vi "Configure Measurement.vi"(0 "Supply Handle in":refnum<k15>, 1 "Active Channel":string, 5 "Supply Measurement Settings":T1={"Measure When Mode"=enum."On Measure Trigger", "Sense Mode"=enum."Local", "Measurement Trigger Terminal"="PXI_Trig0", "Measurement Mode"=enum."Single Point", "Measurement Time (s)"=0.001} {"Measurement Time (s)" format="%#_13p"}, 11 "error in (no error)":errorcluster) -> (4 "Supply Handle out":refnum<k15>, 15 "error out":errorcluster)   [LabVIEW 2018, in "Supply.lvlib"]
uses:
  Supply.lvlib
  Typedefs/Measurement Configuration.ctl
  <instrlib>/niDCPower/nidcpower.llb/niDCPower Configure Digital Edge Measure Trigger.vi
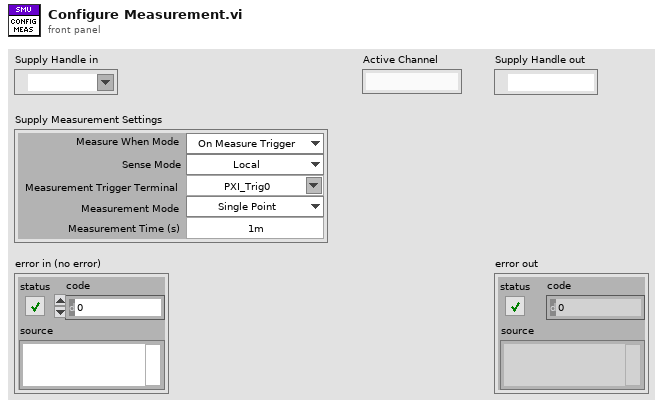
[diagram p1: front panel]
types:
  T1 = typedef "Supply.lvlib/Measurement Configuration.ctl" = cluster{"Measure When Mode":enum16{"Automatically after Source Complete", "On Demand", "On Measure Trigger"}, "Sense Mode":enum16{"Local", "Remote"}, "Measurement Trigger Terminal":string, "Measurement Mode":enum16{"Single Point", "Record"}, "Measurement Time (s)":dbl}
  T2 = enum16{"Automatically after Source Complete", "On Demand", "On Measure Trigger"}
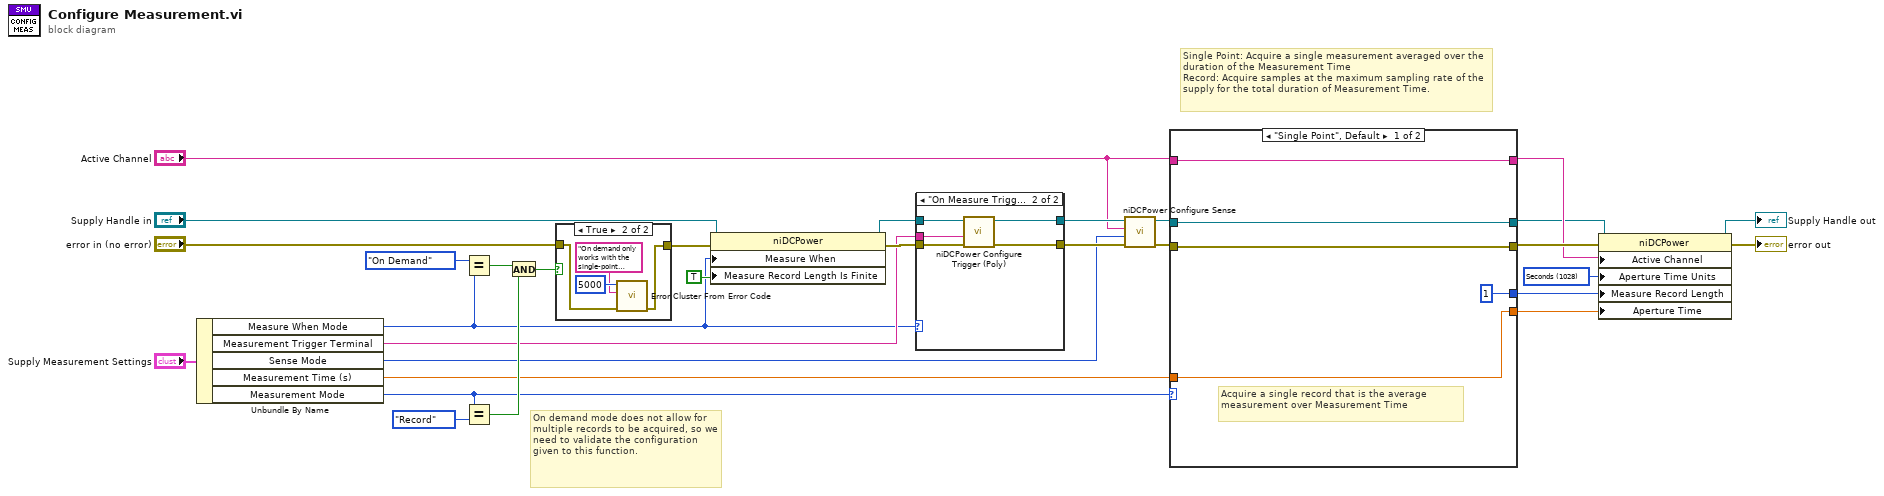
[diagram p0: block diagram]
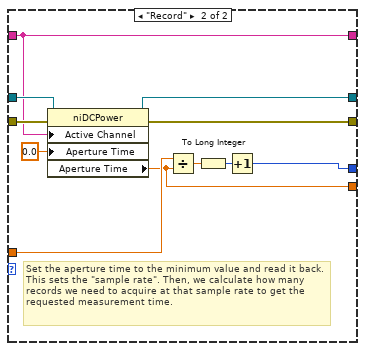
[diagram p4: hidden frame]
diagram:
  w15 = 1028 items=["Seconds"=1028, "Power Line Cycles"=1029] ("Measurement:Aperture Time Units")
  # "Single Point: Acquire a single measurement averaged over the duration of the Measurement Time\nRecord: Acquire samples at the maximum sampling rate of the supply for the total duration of Measurement Time."
  # "On demand mode does not allow for multiple records to be acquired, so we need to validate the configuration given to this function."
  n1 = Unbundle By Name("Supply Measurement Settings") -> ("Measure When Mode"=w7:T2, "Measurement Trigger Terminal"=w24:string, "Sense Mode"=w23:enum16{"Local", "Remote"}, "Measurement Time (s)"=w17:dbl, "Measurement Mode"=w5:enum16{"Single Point", "Record"})
  n2 = Equal?(x=T2."On Demand" ("Measure When Mode"), y=w7) -> (x = y?=w2:bool)
  n3 = Equal?(x=w5, y=enum16{"Single Point", "Record"}."Record" ("Measurement Mode")) -> (x = y?=w30:bool)
  n4 = And(x=w2, y=w30) -> (x .and. y?=w1:bool)
  n5 = case shown="True" w1 {
    tunnel: "error in (no error)" -> [w31 w35]
    tunnel: [w31 w34] -> w3
    frame False {
    }
    frame True {
      n6 = call <vilib>:"Error Cluster From Error Code.vi"("error in (no error)"=w35, "error message (\"\")"="On demand only works with the single-point measurement mode.", "error code (0)"=5000) -> ("error out"=w34:errorcluster)  [unwired: 6 in]
    }
  }
  n7 = property class="niDCPower"(reference="Supply Handle in", error in=w3, "Measure When"=w7, "Measure Record Length Is Finite"=TRUE ("Measurement:Measure Record Length Is Finite")) -> (reference out=w20:refnum<k15>, error out=w26:errorcluster)
  n8 = case shown="\"On Measure Trigger\"" w7 {
    tunnel: [w37 w39] -> w27
    tunnel: w20 -> [w36 w42]
    tunnel: w24 -> [_ w41]
    tunnel: w26 -> [w37 w40]
    tunnel: [w36 w38] -> w25
    frame Default {
    }
    frame "On Measure Trigger" {
      n9 = call-poly <instrlib>:"niDCPower Configure Trigger (Poly).vi"("error in (no error)"=w40, "input terminal"=w41, "instrument handle"=w42) -> ("error out"=w39:errorcluster, "instrument handle out"=w38:refnum<k15>)  [unwired: 7 in]
    }
  }
  n10 = call <instrlib>:"niDCPower Configure Sense.vi"("error in (no error)"=w27, "sense"=w23, "channel name"="Active Channel", "instrument handle"=w25) -> ("error out"=w16:errorcluster, "instrument handle out"=w19:refnum<k15>)  [unwired: 6 in]
  n11 = case shown="\"Single Point\", Default" w5 {
    tunnel: w19 -> [w44 w53]
    tunnel: "Active Channel" -> [w43 w49]
    tunnel: w17 -> [w47 w55]
    tunnel: w16 -> [w45 w54]
    tunnel: [w47 w48] -> w14
    tunnel: [1 ("Measurement:Measure Record Length") w52] -> w13
    tunnel: [w45 w51] -> w12
    tunnel: [w44 w50] -> w8
    tunnel: [w43 w49] -> w9
    frame "Single Point", Default {
      # "Acquire a single record that is the average measurement over Measurement Time"
    }
    frame "Record" {
      # "Set the aperture time to the minimum value and read it back. This sets the \"sample rate\". Then, we calculate how many records we need to acquire at that sample rate to get the requested measurement time."
      n12 = property class="niDCPower"(reference=w53, error in=w54, "Active Channel"=w49, "Aperture Time"=0.0 ("Measurement:Aperture Time")) -> (reference out=w50:refnum<k15>, error out=w51:errorcluster, "Aperture Time"=w48:dbl)
      n13 = Divide(x=w55, y=w48) -> (x/y=w58:dbl)
      n14 = To Long Integer(number=w58) -> (32bit integer=w57:i32)
      n15 = Increment(x=w57) -> (x+1=w52:i32)
    }
  }
  n16 = property class="niDCPower"(reference=w8, error in=w12, "Active Channel"=w9, "Aperture Time Units"=w15, "Measure Record Length"=w13, "Aperture Time"=w14) -> (reference out=→"Supply Handle out":refnum<k15>, error out=→"error out":errorcluster)
